vi "send to python.vi"(8 "waveform":waveform(dbl), 9 "PythonFunctionName":string, 10 "PythonModulePath":path, 11 "Refnum in":refnum<k35>) -> (3 "result":dbl)   [LabVIEW 2020, in "PicoscopeV2.lvclass"]
uses:
  PicoscopeV2.lvclass
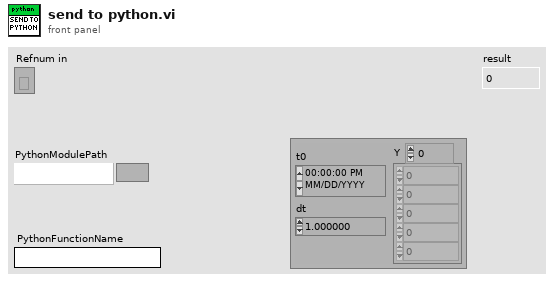
[diagram p1: front panel]
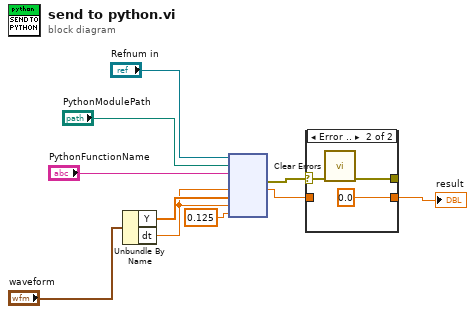
[diagram p0: block diagram]
diagram:
  n1 = Unbundle By Name("waveform") -> ("Y"=w6:dbl[], "dt"=w4:dbl)
  n2 = node("Refnum in", "PythonModulePath", "PythonFunctionName", w4, w6, w4, 0.125 ("Numeric")) -> (w3:errorcluster, w2:dbl)  [unwired: 4 in, 3 out]
  n3 = case shown="Error .." w3 {
    selector: w3 -> [w11 w14]
    tunnel: w2 -> [w12 _]
    tunnel: [w12 0.0 ("dt")] -> w10
    tunnel: [w11 w13] -> _
    frame No Error {
    }
    frame Error {
      n4 = call <vilib>:"Clear Errors.vi"("error in (no error)"=w14) -> ("error out"=w13:errorcluster)  [unwired: 5 in, 1 out]
    }
  }
  "result" <- w10
